vi "getSettings.vi"(7 "LabVIEW Web Service Request":refnum<class "Web Request.lvclass">, 10 "reservation_id":string, 11 "context_id":string) -> (2 "back_url":string, 3 "base_url":string)   [LabVIEW 2013]
uses:
  <vilib>/wsapi/Web Request.lvclass
  <vilib>/Utility/config.llb/Read Key (String).vi
  <vilib>/Utility/config.llb/NI_LVConfig.lvlib
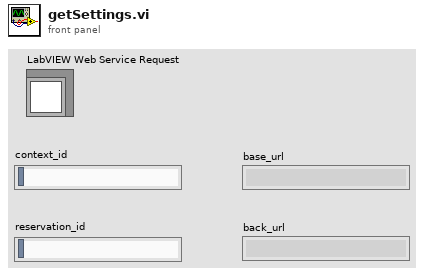
[diagram p1: front panel]
types:
  T1 = typedef "NI_LVConfig.lvlib/Config Data RefNum.ctl" = refnum<k1>
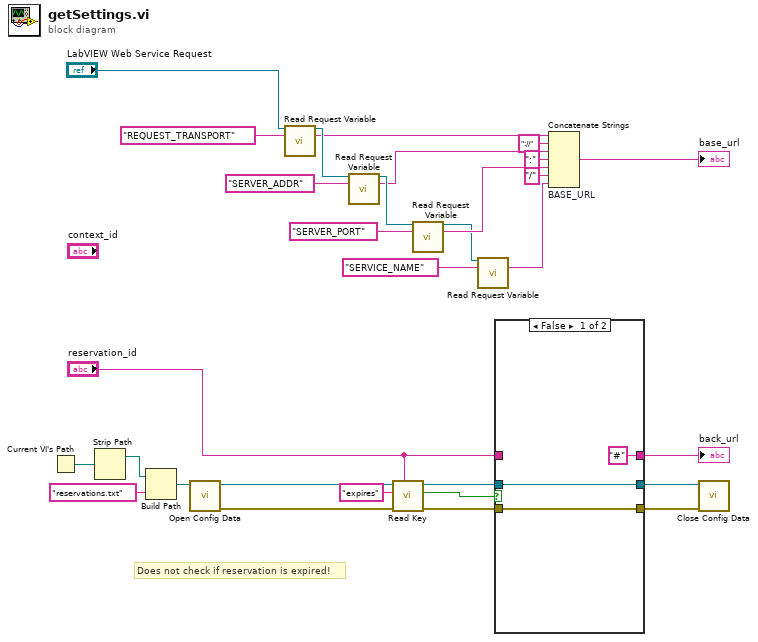
[diagram p0: block diagram]
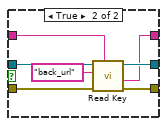
[diagram p2: hidden frame]
diagram:
  # "Does not check if reservation is expired!"
  n1 = Current VI's Path() -> (path=w30:path)
  n2 = Strip Path(path=w30) -> (stripped path=w29:path)  [unwired: 1 out]
  n3 = Build Path(base path=w29, name or relative path="reservations.txt") -> (appended path=w27:path)
  n4 = call <vilib>:"Open Config Data.vi"("configuration file path"=w27) -> ("error out"=w24:errorcluster, "refnum"=w25:T1)  [unwired: 8 in, 1 out]
  n5 = call <vilib>:"Read Request Variable.vi"("LabVIEW Web Service Request"="LabVIEW Web Service Request", "variable name"="REQUEST_TRANSPORT") -> ("LabVIEW Web Service Request out"=w16:refnum<class "Web Request.lvclass">, "value"=w14:string)  [unwired: 11 in, 1 out]
  n6 = call <vilib>:"Read Request Variable.vi"("LabVIEW Web Service Request"=w16, "variable name"="SERVER_ADDR") -> ("LabVIEW Web Service Request out"=w15:refnum<class "Web Request.lvclass">, "value"=w12:string)  [unwired: 11 in, 1 out]
  n7 = call-poly <vilib>:"Read Key.vi"("section"="reservation_id", "error in (no error)"=w24, "key"="expires", "refnum"=w25) -> ("error out"=w21:errorcluster, "found?"=w23:bool, "refnum out"=w22:T1)  [unwired: 4 in, 1 out]
  n8 = call <vilib>:"Read Request Variable.vi"("LabVIEW Web Service Request"=w15, "variable name"="SERVER_PORT") -> ("LabVIEW Web Service Request out"=w7:refnum<class "Web Request.lvclass">, "value"=w10:string)  [unwired: 11 in, 1 out]
  n9 = call <vilib>:"Read Request Variable.vi"("LabVIEW Web Service Request"=w7, "variable name"="SERVICE_NAME") -> ("value"=w4:string)  [unwired: 11 in, 2 out]
  n10 = case shown="False" w23 {
    tunnel: w22 -> [w33 w40]
    tunnel: w21 -> [w32 w39]
    tunnel: "reservation_id" -> [_ w38]
    tunnel: [w33 w36] -> w3
    tunnel: [w32 w35] -> w2
    tunnel: ["#" ("value") w34] -> w1
    frame False {
    }
    frame True {
      n11 = call-poly <vilib>:"Read Key.vi"("section"=w38, "error in (no error)"=w39, "key"="back_url", "refnum"=w40) -> ("error out"=w35:errorcluster, "value"=w34:string, "refnum out"=w36:T1)  [unwired: 4 in, 1 out]
    }
  }
  "back_url" <- w1
  n12 = Concatenate Strings "BASE_URL"(w14, "://" ("string"), w12, ":" ("string"), w10, "/" ("string"), w4) -> (→"base_url":string)
  n13 = call <vilib>:"Close Config Data.vi"("error in (no error)"=w2, "refnum"=w3) -> ()  [unwired: 8 in, 2 out]
